vi "Flatten.vi"(8 "error in (no error)":errorcluster, 9 "FIFO Timestamps":T1, 10 "Data in":u8[](array[numeric]) format="%.0x", 11 "CIFfifo in":refnum<class "CIFfifo.lvclass">) -> (0 "error out":errorcluster, 3 "CIFfifo out":refnum<class "CIFfifo.lvclass">)   [LabVIEW 2021, in "CIFfifo.lvclass"]
uses:
  CIFfifo.lvclass
  CIFfifo.lvclass/CIFfifo.ctl
  ChannelCommon.lvlib
  typedef/TimeStamps.ctl
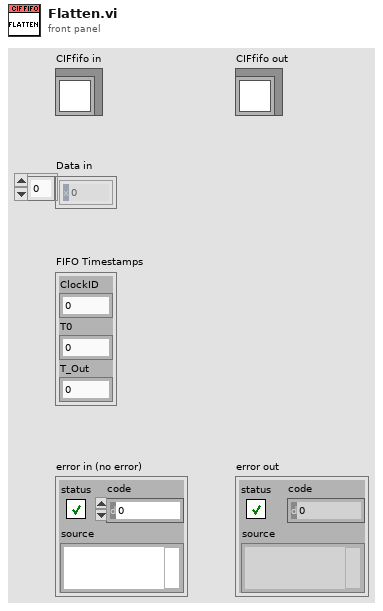
[diagram p1: front panel]
types:
  T1 = typedef "ChannelCommon.lvlib/TimeStamps.ctl" = cluster{"ClockID":u8, "T0":i64, "T_Out":i64}
  T2 = typedef "ChannelCommon.lvlib/FIFO Header.ctl" = cluster{"Length":u64, "T0":i64, "T_Out":i64, "T_Tx":i64, "Ctr":u64, "ClockID":u8}
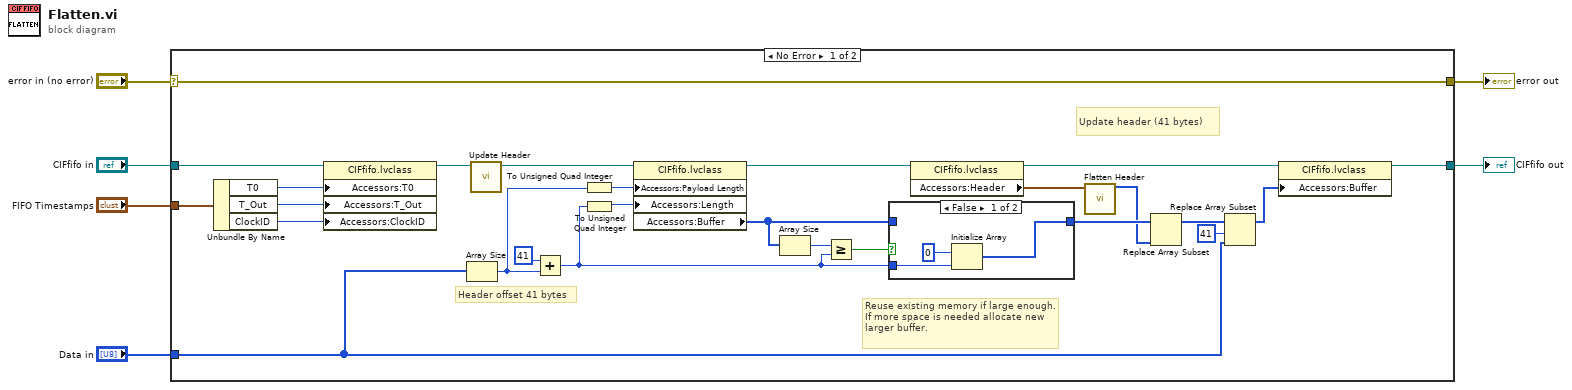
[diagram p0: block diagram]
diagram:
  n1 = case shown="No Error" "error in (no error)" {
    selector: "error in (no error)" -> [w14 w38]
    tunnel: [w14 w38] -> w1
    tunnel: [w10 w37] -> w2
    tunnel: "CIFfifo in" -> [w27 w37]
    tunnel: "FIFO Timestamps" -> [w32 _]
    tunnel: "Data in" -> [w26 _]
    frame No Error {
      # "Header offset 41 bytes"
      # "Update header (41 bytes)"
      # "Reuse existing memory if large enough.  If more space is needed allocate new larger buffer."
      n2 = Unbundle By Name(w32) -> ("T0"=w28:i64, "T_Out"=w29:i64, "ClockID"=w30:u8)
      n3 = property class="CIFfifo.lvclass"(reference=w27, "Accessors:T0"=w28, "Accessors:T_Out"=w29, "Accessors:ClockID"=w30) -> (reference out=w31:refnum<class "CIFfifo.lvclass">)  [unwired: 1 in, 1 out]
      n4 = Array Size(array=w26) -> (size(s)=w19:i32)
      n5 = call "Update Header.vi"("CIFFIFO in"=w31) -> ("CIFFIFO out"=w13:refnum<class "CIFfifo.lvclass">)  [unwired: 10 in]
      n6 = Add(x=41 ("y"), y=w19) -> (x+y=w7:i32)
      n7 = To Unsigned Quad Integer(1:w19) -> (0:w24:u64)
      n8 = To Unsigned Quad Integer(1:w7) -> (0:w9:u64)
      n9 = property class="CIFfifo.lvclass"(reference=w13, "Accessors:Payload Length"=w24, "Accessors:Length"=w9) -> (reference out=w21:refnum<class "CIFfifo.lvclass">, "Accessors:Buffer"=w8:u8[])  [unwired: 1 in, 1 out]
      n10 = Array Size(array=w8) -> (size(s)=w23:i32)
      n11 = Greater Or Equal?(x=w23, y=w7) -> (x >= y?=w22:bool)
      n12 = case shown="False" w22 {
        tunnel: w8 -> [_ w36]
        tunnel: [w33 w36] -> w18
        tunnel: w7 -> [w35 _]
        frame False {
          n13 = Initialize Array(u8 0, w35) -> (w33:u8[])
        }
        frame True {
        }
      }
      n14 = property class="CIFfifo.lvclass"(reference=w21) -> (reference out=w12:refnum<class "CIFfifo.lvclass">, "Accessors:Header"=w25:T2)  [unwired: 1 in, 1 out]
      n15 = call "Flatten Header.vi"("Header in"=w25) -> ("Flattened Data out"=w17:u8[])  [unwired: 10 in]
      n16 = Replace Array Subset(array=w18, new element=w17) -> (w16:u8[])  [unwired: 1 in]
      n17 = Replace Array Subset(array=w16, new element=w26, index=41) -> (w11:u8[])
      n18 = property class="CIFfifo.lvclass"(reference=w12, "Accessors:Buffer"=w11) -> (reference out=w10:refnum<class "CIFfifo.lvclass">)  [unwired: 1 in, 1 out]
    }
    frame Error {
    }
  }
  "error out" <- w1
  "CIFfifo out" <- w2
